vi "DownloadFile.vi"(8 "error in (no error)":errorcluster, 10 "file":path=path "/Kim/Users/crogers/Desktop/SRV/srv1.ldr", 11 "SRV In":refnum<k5>) -> (0 "error out":errorcluster, 3 "SRV Out":refnum<k5>)   [LabVIEW 2009]
doc: "Downloads a file to the SRV.\n\nModifed for Benilde St. Margaret's School - Tim Jump\nBy Doug Schmertman - Logic PD\nCopyright 2012"
panel:
  # "This LabVIEW item is deprecated.\n\nIt is believed to be unused and will be removed in a future version of SRV."
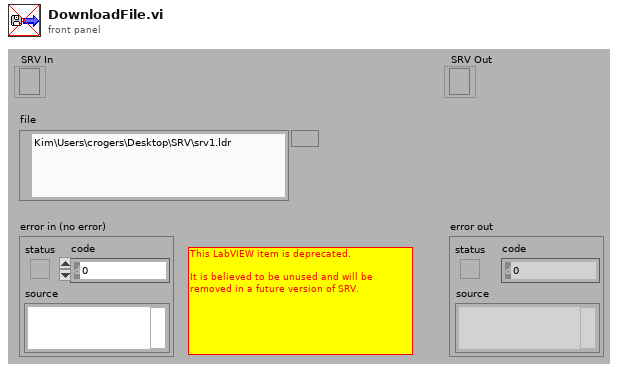
[diagram p1: front panel]
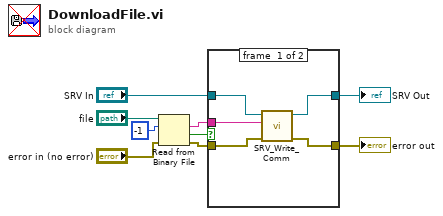
[diagram p0: block diagram]
diagram:
  n1 = Read from Binary File(8:"error in (no error)", 10:-1 ("count (1)"), 11:"file") -> (0:w2:errorcluster, 1:w6:bool, 2:w7:string)  [unwired: 3 in, 1 out]
  n2 = case shown="False" w6 {
    tunnel: "SRV In" -> [w14 w16]
    tunnel: [w13 w16] -> w4
    tunnel: w7 -> [w12 _]
    tunnel: w2 -> [w11 w15]
    tunnel: [w10 w15] -> w1
    frame #0 {
      n3 = call "SRV_Write_Comm.vi"("error in (no error)"=w11, "Command Sent"=w12, "SRV In"=w14) -> ("error out"=w10:errorcluster, "SRV Out"=w13:refnum<k5>)  [unwired: 6 in, 1 out]
    }
    frame #1 {
    }
  }
  "SRV Out" <- w4
  "error out" <- w1
